vi "myRIO__TCP_constants_byteRange_numbers.vi"() -> (1 "output_byte_end":u8=57, 3 "output_byte_start":u8=48, 4 "output_byte_negativeSign":u8=57)   [LabVIEW 2014]
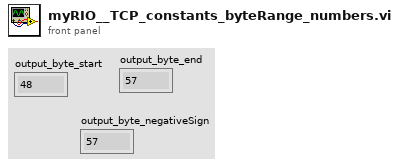
[diagram p1: front panel]
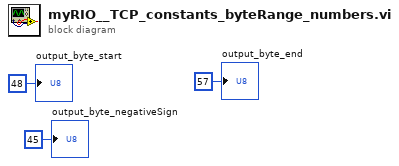
[diagram p0: block diagram]
diagram:
  "output_byte_end" <- u8 57
  "output_byte_start" <- u8 48
  "output_byte_negativeSign" <- u8 45 ("output_byte_end 2")
